vi "Get Protocol Type.vi"(8 "error in (no error)":errorcluster, 11 "AK TCP in":refnum<class "AK TCP.lvclass">) -> (0 "error out":errorcluster, 2 "protocol type":T1=enum."AK RS-XXX", 3 "AK TCP out":refnum<class "AK TCP.lvclass">)   [LabVIEW 2023, in "Protocols.lvlib" / "AK TCP.lvclass"]
doc: "Returns AK TCP|IP protocol type Enum."
uses:
  AK TCP.lvclass
  Protocol Parent/Types/Protocol Type.ctl
  Protocol Parent/Protocol Parent.lvclass
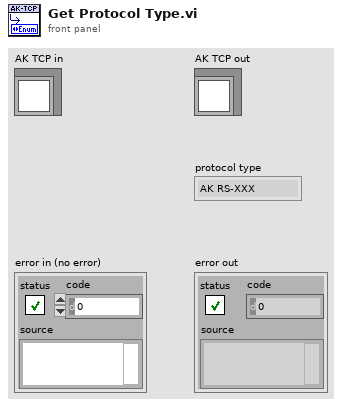
[diagram p1: front panel]
types:
  T1 = typedef "Protocols.lvlib/Protocol Parent.lvclass/Protocol Type.ctl" = enum16{"RS-XXX", "AK RS-XXX", "VISA", "TCPIP", "AK TCPIP", "UDP", "GPIB ConvBox"}
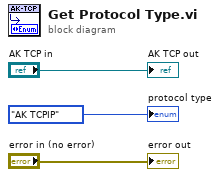
[diagram p0: block diagram]
diagram:
  "error out" <- "error in (no error)"
  "AK TCP out" <- "AK TCP in"
  "protocol type" <- Protocol_Type."AK TCPIP" ("Protocol out")
